vi "StopMeas.vi"(8 "error in (no error)":errorcluster, 11 "NHRDCPower in":refnum<class "NHRDCPower.lvclass">) -> (0 "error out":errorcluster, 3 "NHRDCPower out":refnum<class "NHRDCPower.lvclass">)   [LabVIEW 2018, in "AcPwrPlugins.lvlib" / "NHRDCPower.lvclass"]
doc: "This VI stops the measurements."
uses:
  NHRDCPower.lvclass
  <instrlib>/NHRDCPowerModule/NHRDCPowerModule/NHRDCPowerModule.lvlib
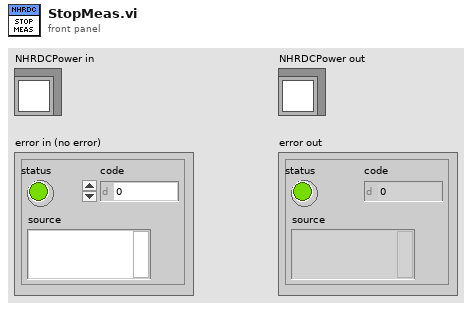
[diagram p1: front panel]
types:
  T1 = typedef "AcPwrPlugins.lvlib/NHRDCPower.lvclass/Measurements.ctl" = cluster{"Handle":string, "Name":string, "Enabled":bool, "Measurement Value":sgl, "Measurement Type":enum16{"Power", "Current", "Voltage"}}[]
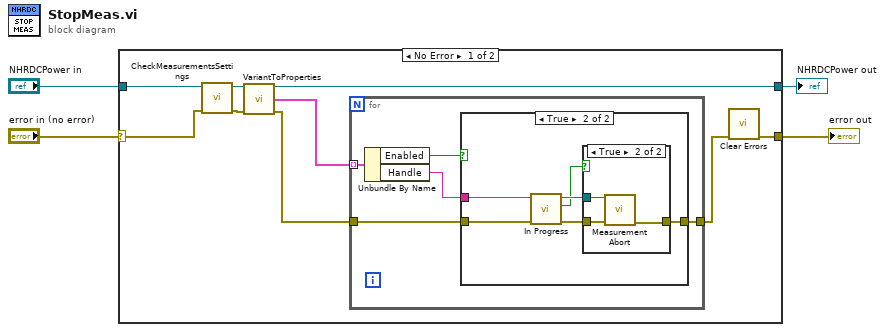
[diagram p0: block diagram]
diagram:
  n1 = case shown="No Error" "error in (no error)" {
    selector: "error in (no error)" -> [w8 w30]
    tunnel: [w5 w30] -> w1
    tunnel: [w6 w31] -> w2
    tunnel: "NHRDCPower in" -> [w10 w31]
    frame No Error {
      n2 = call-dynamic "CheckMeasurementsSettings.vi"("error in (no error)"=w8, "NHRDCPower in"=w10) -> ("error out"=w12:errorcluster, "NHRDCPower out"=w11:refnum<class "NHRDCPower.lvclass">)  [unwired: 8 in]
      n3 = call "VariantToProperties.vi"("NHRDCPower in"=w11, "error in (no error)"=w12) -> ("NHRDCPower out"=w6:refnum<class "NHRDCPower.lvclass">, "Meas"=w9:T1, "error out"=w7:errorcluster)  [unwired: 7 in, 4 out]
      n4 = for {
        tunnel: w9 -> [w18] mode=indexing
        tunnel: w7 -> [w17]
        tunnel: [w16] -> w13
        n5 = Unbundle By Name(w18) -> ("Enabled"=w15:bool, "Handle"=w14:string)
        n6 = case shown="True" w15 {
          tunnel: w17 -> [w19 w24]
          tunnel: [w19 w25] -> w16
          tunnel: w14 -> [_ w21]
          frame False {
          }
          frame True {
            n7 = call <instrlib>:"In Progress.vi"("error in (no error)"=w24, "instrument handle"=w21) -> ("error out"=w23:errorcluster, "in progress"=w20:bool, "instrument handle out"=w22:refnum<visa-resource-name>)  [unwired: 7 in]
            n8 = case shown="True" w20 {
              tunnel: w23 -> [w26 w29]
              tunnel: [w26 w27] -> w25
              tunnel: w22 -> [_ w28]
              frame False {
              }
              frame True {
                n9 = call <instrlib>:"Measurement Abort.vi"("error in (no error)"=w29, "instrument handle"=w28) -> ("error out"=w27:errorcluster)  [unwired: 8 in, 1 out]
              }
            }
          }
        }
      }
      n10 = call <vilib>:"Clear Errors.vi"("error in (no error)"=w13) -> ("error out"=w5:errorcluster)  [unwired: 5 in, 1 out]
    }
    frame Error {
    }
  }
  "error out" <- w1
  "NHRDCPower out" <- w2
